vi "获取溶解氧监测值.vi"(8 "error in (no error)":errorcluster caption="错误输入（无错误）") -> (0 "error out":errorcluster caption="错误输出", 3 "监测值":T1)   [LabVIEW 2016, in "NAQ_DO.lvlib"]
uses:
  NAQ_DO.lvlib
  <vilib>/Plasmionique/MB Master/MB_Master/MB_Master.lvclass
  elevator/elevator.lvlib
  <vilib>/Plasmionique/MB Master/MB Master.lvlib
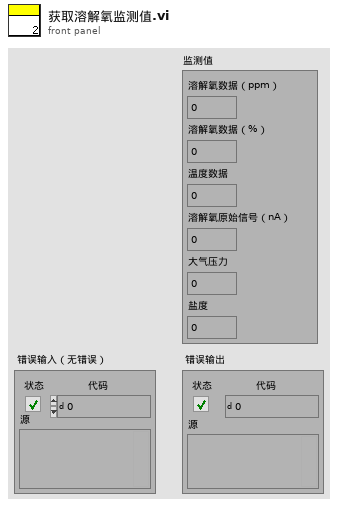
[diagram p1: front panel]
types:
  T1 = cluster{"溶解氧数据（ppm）":dbl, "溶解氧数据（%）":dbl, "温度数据":dbl, "溶解氧原始信号（nA）":dbl, "大气压力":dbl, "盐度":dbl}
  T2 = cluster{"数组 2[0]":sgl, "数组 2[1]":sgl, "数组 2[2]":sgl, "数组 2[3]":sgl, "数组 2[4]":sgl, "数组 2[5]":sgl}
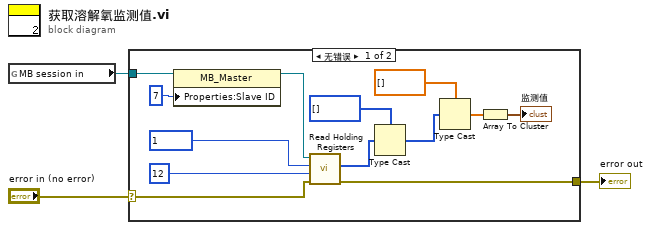
[diagram p0: block diagram]
diagram:
  n1 = global read "elevator 全局变量.vi" "MB session in"() -> (w1:refnum<class "MB_Master.lvclass">)
  n2 = case shown="无错误" "error in (no error)" {
    selector: "error in (no error)" -> [w12 w17]
    tunnel: [w16 w17] -> w3
    tunnel: w1 -> [w11 _]
    frame No Error {
      n3 = property class="MB_Master"(reference=w11, "Properties:Slave ID"=7) -> (reference out=w14:refnum<class "MB_Master.lvclass">)  [unwired: 1 in, 1 out]
      n4 = call <vilib>:"Read Holding Registers.vi"("error in (no error)"=w12, "quantity"=u16 12, "starting address"=u16 1, "MB session in"=w14) -> ("error out"=w16:errorcluster, "Registers"=w6:u16[])  [unwired: 5 in, 1 out]
      n5 = Type Cast(type=u32[] [] ("数组 2"), x=w6) -> (*(type *) &x=w9:u32[])
      n6 = Type Cast(type=sgl[] [] ("数组 2"), x=w9) -> (*(type *) &x=w5:sgl[])
      n7 = Array To Cluster(array=w5) -> (cluster=→"监测值":T2)
    }
    frame Error {
    }
  }
  "error out" <- w3
